vi "RANGE Update Averages.vi"(0 "DAQ Data Out in":T1, 1 "Average Updates":T1, 5 "Error In":errorcluster, 6 "Meter Bank 1.Start ANSI":bool, 7 "Gas Mix Number Bank 1":string="240", 8 "Meter Bank 2.Start ANSI":bool, 9 "Gas Mix Number Bank 2":string="241", 10 "Meter Bank 3.Start ANSI":bool, 11 "Gas Mix Number Bank 3":string="242") -> (14 "DAQ Data Out out":T1, 19 "Error Out":errorcluster)   [LabVIEW 2016]
uses:
  Type Definitions/RANGE DAQ Data Four Meters.ctl
  Type Definitions/RANGE DAQ Data.ctl
  Drivers/Omega FMA-1600A Series Gas Flow Meter/Type Definitions/FMA1600A Gas Type.ctl
  Drivers/Omega FMA-1600A Series Gas Flow Meter/Type Definitions/FMA1600A Units String.ctl
  Type Definitions/RANGE GAS Data.ctl
  Type Definitions/RANGE Panel Data.ctl
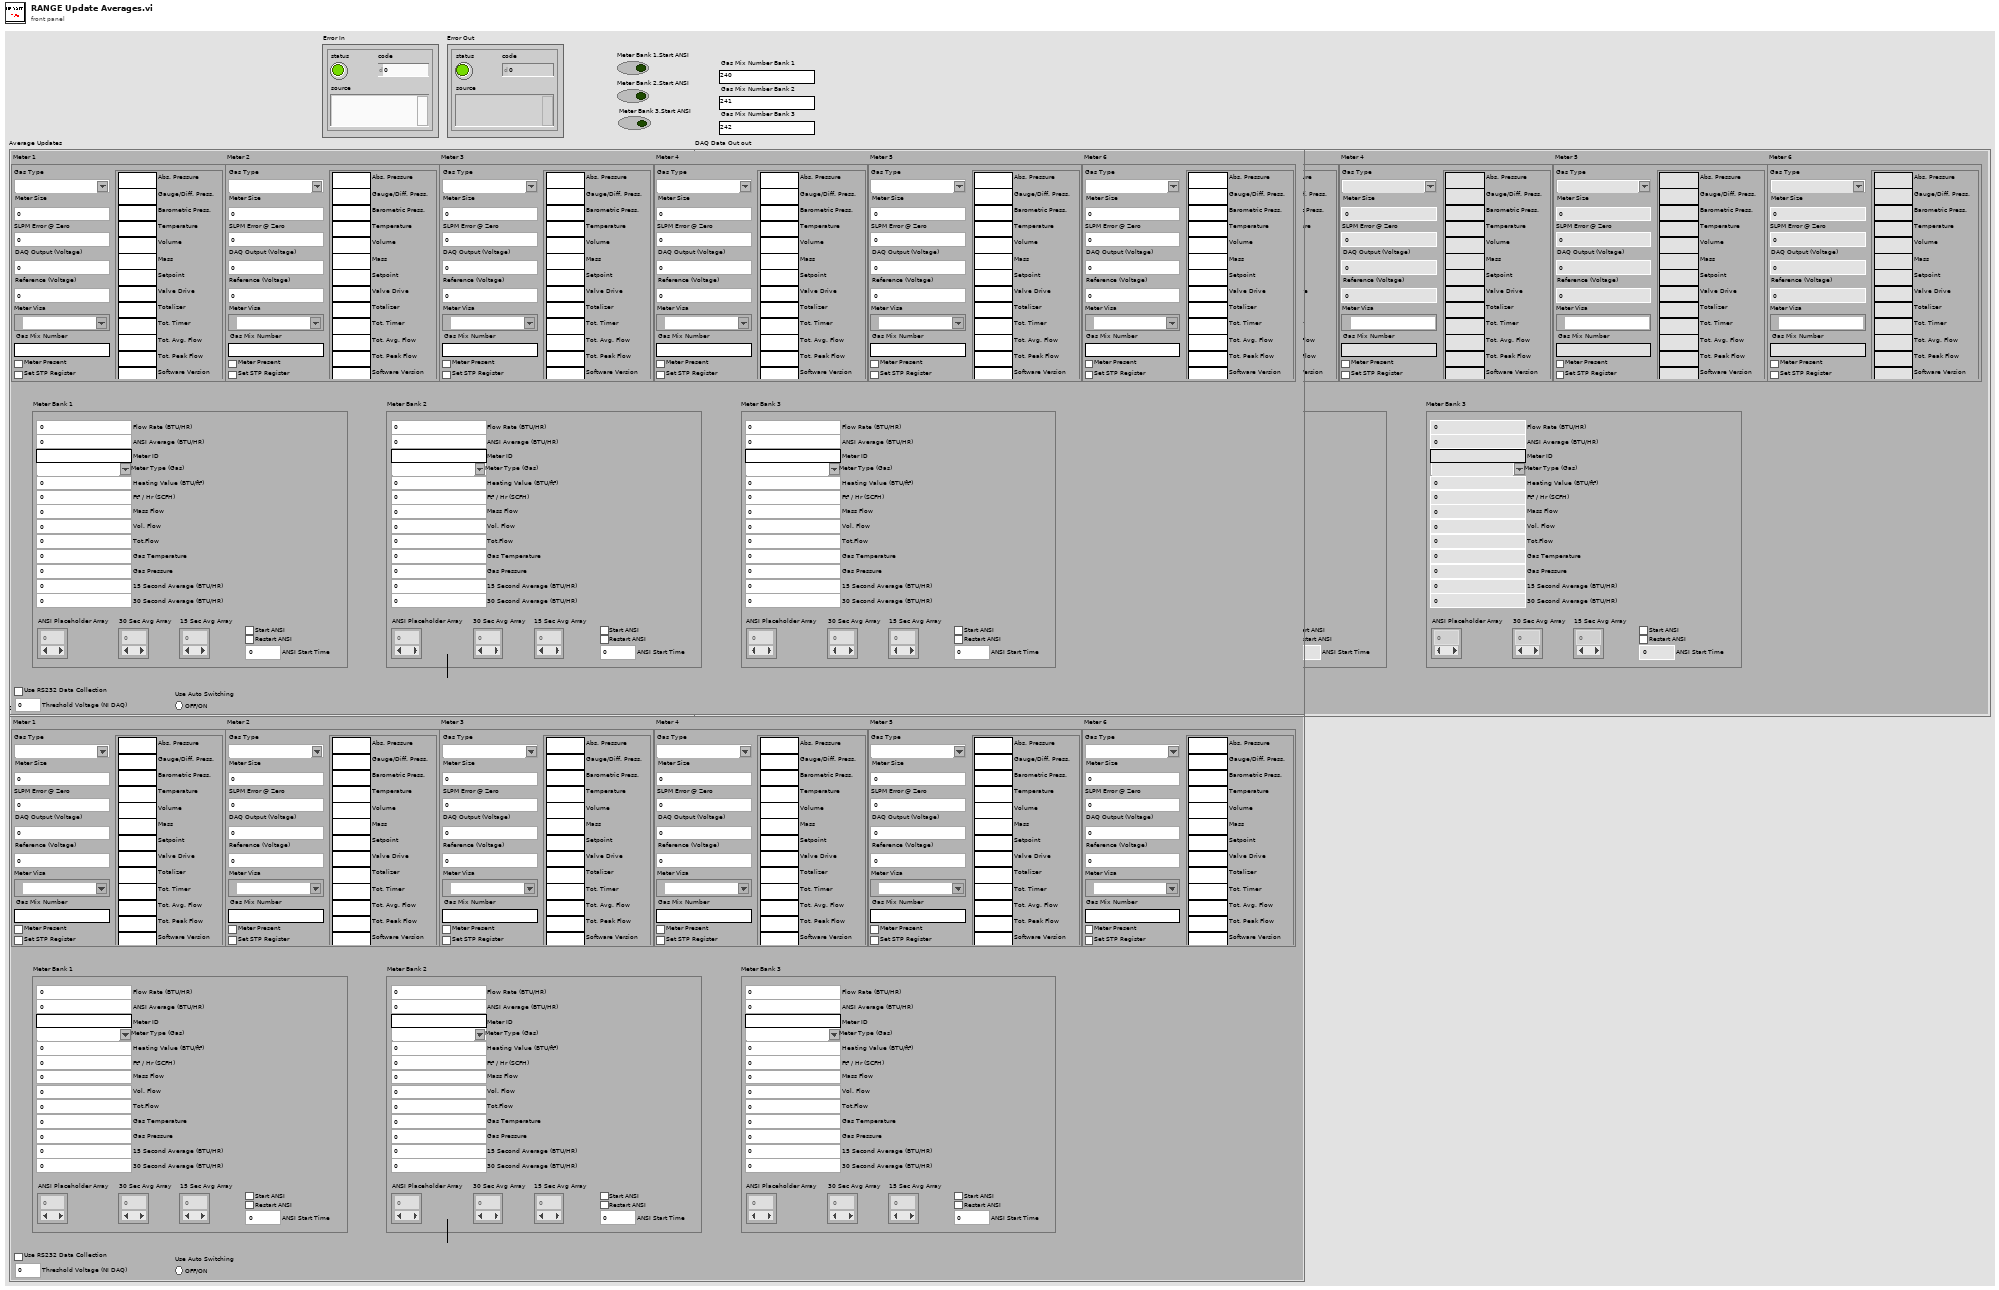
[diagram p1: front panel]
types:
  T1 = typedef "RANGE DAQ Data Four Meters.ctl" = cluster{"Meter 1":T2, "Meter 2":T2, "Meter 3":T2, "Meter 4":T2, "Meter 5":T2, "Meter 6":T2, "Meter Bank 1":T5, "Meter Bank 2":T5, "Meter Bank 3":T5, "Threshold Voltage (NI DAQ)":dbl, "Use RS232 Data Collection":bool, "Use Auto Switching":bool}
  T2 = typedef "RANGE DAQ Data.ctl" = cluster{"Meter Size":dbl, "DAQ Output (Voltage)":dbl, "Reference (Voltage)":dbl, "Meter Present":bool, "Meter Visa":refnum<visa-resource-name>, "Gas Type":T3, "SLPM Error @ Zero":dbl, "Gas Mix Number":string, "Set STP Register":bool, "Measurement Units":T4}
  T3 = typedef "FMA1600A Gas Type.ctl" = string
  T4 = typedef "FMA1600A Units String.ctl" = cluster{"Abs. Pressure":string, "Gauge/Diff. Press.":string, "Barometric Press.":string, "Temperature":string, "Volume":string, "Mass":string, "Setpoint":string, "Valve Drive":string, "Totalizer":string, "Tot. Timer":string, "Tot. Avg. Flow":string, "Tot. Peak Flow":string, "Software Version":string}
  T5 = typedef "RANGE GAS Data.ctl" = cluster{"Flow Rate (BTU/HR)":dbl, "ANSI Placeholder Array":dbl[], "15 Sec Avg Array":dbl[], "30 Sec Avg Array ":dbl[], "ANSI Average (BTU/HR)":dbl, "Panel Data":T6, "Start ANSI":bool, "ANSI Start Time":dbl, "Restart ANSI":bool, "Meter ID":string}
  T6 = typedef "RANGE Panel Data.ctl" = cluster{"Meter Type (Gas)":T3, "Heating Value (BTU/ft³)":dbl, "Ft³ / Hr (SCFH)":dbl, "15 Second Average (BTU/HR)":dbl, "30 Second Average (BTU/HR)":dbl, "Mass Flow":dbl, "Vol. Flow":dbl, "Gas Temperature":dbl, "Gas Pressure":dbl, "Tot.Flow":dbl}
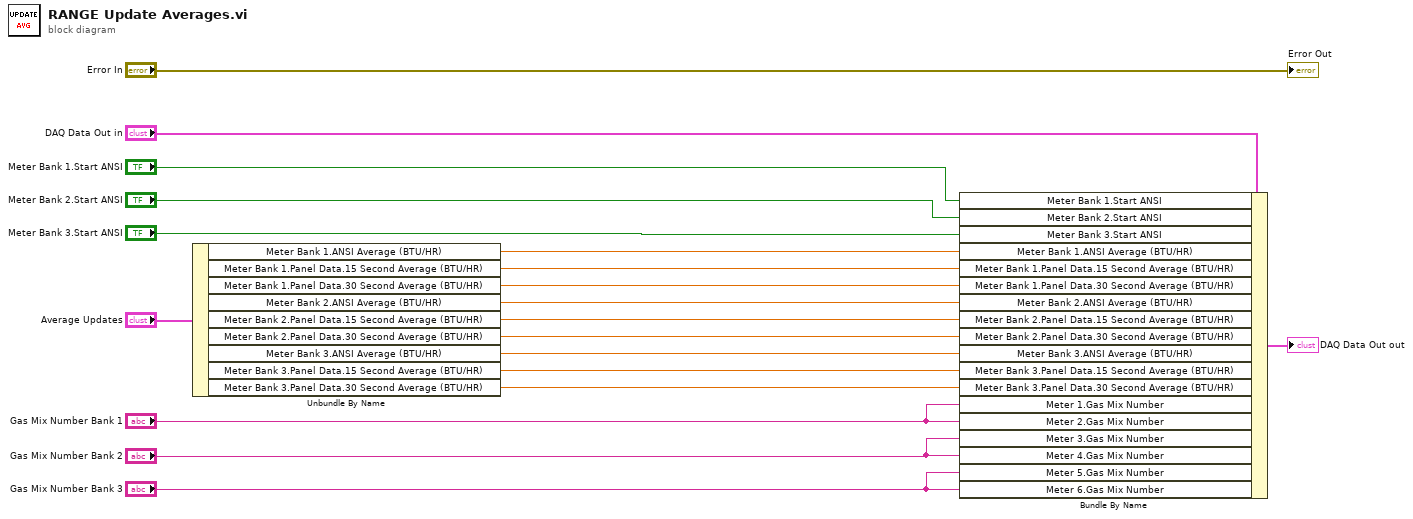
[diagram p0: block diagram]
diagram:
  n1 = Unbundle By Name("Average Updates") -> ("Meter Bank 1.ANSI Average (BTU/HR)"=w18:dbl, "Meter Bank 1.Panel Data.15 Second Average (BTU/HR)"=w17:dbl, "Meter Bank 1.Panel Data.30 Second Average (BTU/HR)"=w16:dbl, "Meter Bank 2.ANSI Average (BTU/HR)"=w15:dbl, "Meter Bank 2.Panel Data.15 Second Average (BTU/HR)"=w14:dbl, "Meter Bank 2.Panel Data.30 Second Average (BTU/HR)"=w13:dbl, "Meter Bank 3.ANSI Average (BTU/HR)"=w12:dbl, "Meter Bank 3.Panel Data.15 Second Average (BTU/HR)"=w11:dbl, "Meter Bank 3.Panel Data.30 Second Average (BTU/HR)"=w10:dbl)
  n2 = Bundle By Name(cluster="DAQ Data Out in", "Meter Bank 1.Start ANSI"="Meter Bank 1.Start ANSI", "Meter Bank 2.Start ANSI"="Meter Bank 2.Start ANSI", "Meter Bank 3.Start ANSI"="Meter Bank 3.Start ANSI", "Meter Bank 1.ANSI Average (BTU/HR)"=w18, "Meter Bank 1.Panel Data.15 Second Average (BTU/HR)"=w17, "Meter Bank 1.Panel Data.30 Second Average (BTU/HR)"=w16, "Meter Bank 2.ANSI Average (BTU/HR)"=w15, "Meter Bank 2.Panel Data.15 Second Average (BTU/HR)"=w14, "Meter Bank 2.Panel Data.30 Second Average (BTU/HR)"=w13, "Meter Bank 3.ANSI Average (BTU/HR)"=w12, "Meter Bank 3.Panel Data.15 Second Average (BTU/HR)"=w11, "Meter Bank 3.Panel Data.30 Second Average (BTU/HR)"=w10, "Meter 1.Gas Mix Number"="Gas Mix Number Bank 1", "Meter 2.Gas Mix Number"="Gas Mix Number Bank 1", "Meter 3.Gas Mix Number"="Gas Mix Number Bank 2", "Meter 4.Gas Mix Number"="Gas Mix Number Bank 2", "Meter 5.Gas Mix Number"="Gas Mix Number Bank 3", "Meter 6.Gas Mix Number"="Gas Mix Number Bank 3") -> (→"DAQ Data Out out":T1)
  "Error Out" <- "Error In"
